vi "RG Get User Input Wavelength.vi"(9 "Current wavelength":dbl format="%#_13g") -> (1 "Cancelled?":bool, 2 "Go to wavelength":dbl)   [LabVIEW 2017, in "Monochromator.lvlib"]
uses:
  Monochromator.lvlib
panel:
  out "concatenated string":string
  in  "Cancel":bool
  in  "OK":bool
  in  "Move to wavelength?":string
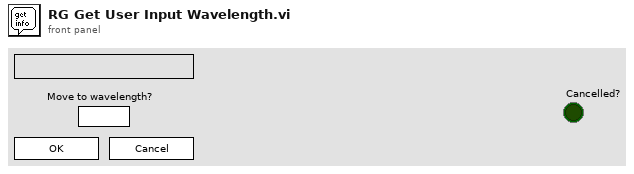
[diagram p1: front panel]
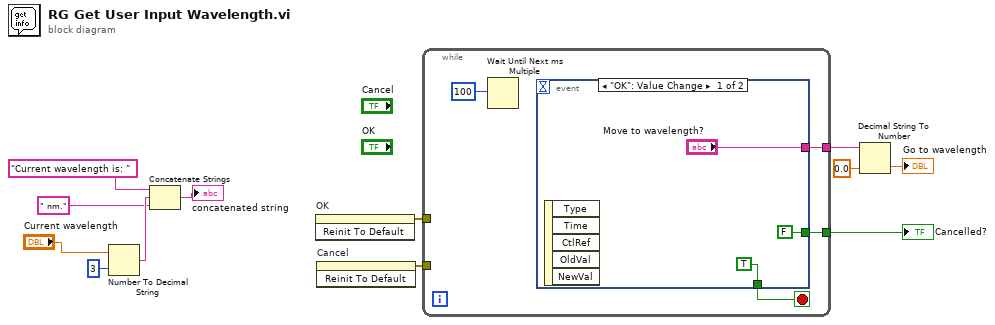
[diagram p0: block diagram]
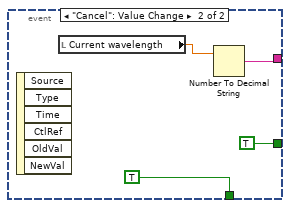
[diagram p2: hidden frame]
diagram:
  n1 = Number To Decimal String(number="Current wavelength", width (-)=i16 3) -> (decimal integer string=w5:string)
  n2 = Concatenate Strings("Current wavelength is: " ("String"), w5, " nm." ("string")) -> (→"concatenated string":string)
  n3 = invoke on="OK" class="Bool" method="Reinit To Default"() -> (error out=w12:errorcluster)  [unwired: 3 in, 2 out]
  n4 = invoke on="Cancel" class="Bool" method="Reinit To Default"() -> (error out=w11:errorcluster)  [unwired: 3 in, 2 out]
  n5 = while {
    tunnel: [w16] -> w10
    tunnel: w12 -> [_]
    tunnel: w11 -> [_]
    tunnel: [w13] -> w1
    stop <- w14 stop-if-true
    n6 = Wait Until Next ms Multiple(millisecond multiple=100) -> ()  [unwired: 1 out]
    n7 = event shown="[0] \"OK\": Value Change" {
      selector: _ -> [_ _]
      dyn-events: _ -> [_ _]
      timeout: _ -> [_ _]
      tunnel: [TRUE TRUE] -> w14
      tunnel: ["Move to wavelength?" w22] -> w16
      tunnel: [FALSE TRUE] -> w13
      event "OK": Value Change {
        n8 = event-data() -> ()  [unwired: 6 out]
      }
      event "Cancel": Value Change {
        n9 = event-data() -> ()  [unwired: 7 out]
        n10 = local read "Current wavelength"() -> (w21:dbl)
        n11 = Number To Decimal String(number=w21) -> (decimal integer string=w22:string)  [unwired: 1 in]
      }
    }
  }
  "Cancelled?" <- w1
  n12 = Decimal String To Number(string=w10, default (0L)=0.0 ("default (0 I32)")) -> (number=→"Go to wavelength":dbl)  [unwired: 1 in, 1 out]
